vi "WaterVapourSaturationPressure.vi"(1 "Temperature (K)":dbl) -> (0 "Water Vapour Saturation Pressure (Pa)":dbl)   [LabVIEW 2014]
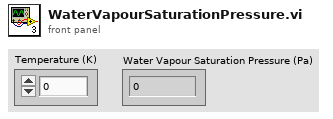
[diagram p1: front panel]
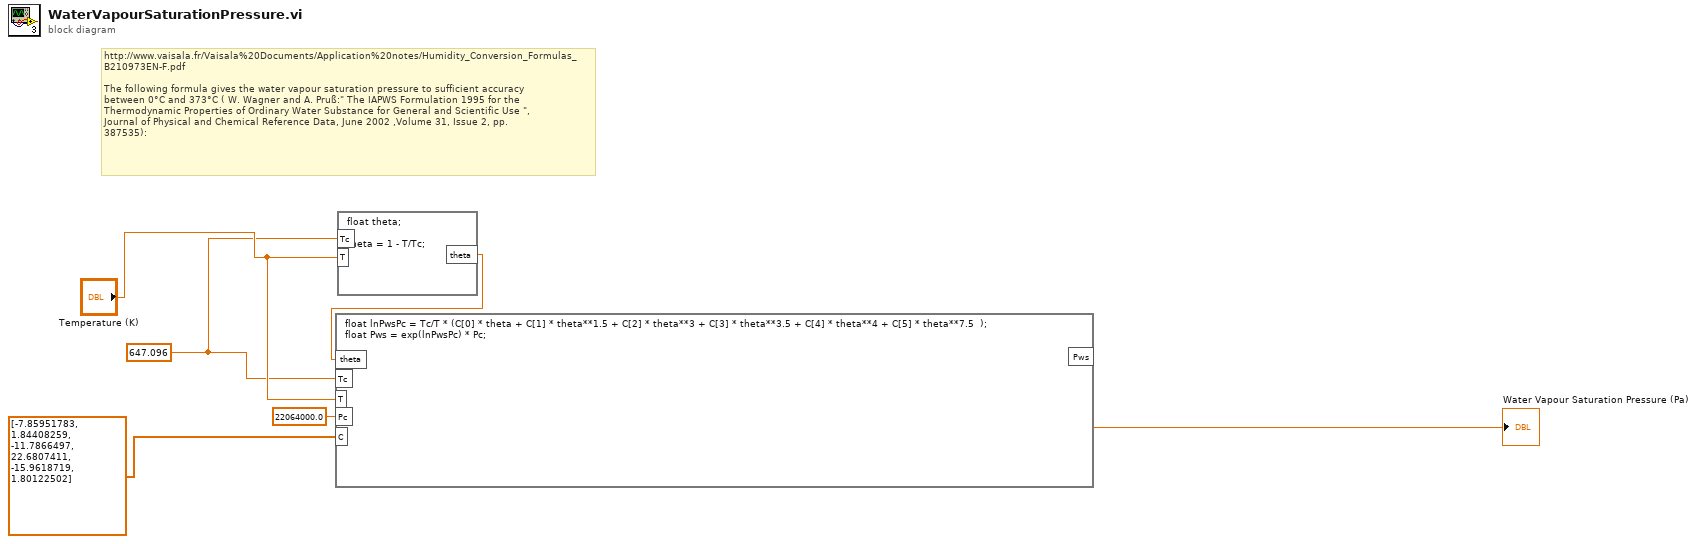
[diagram p0: block diagram]
diagram:
  w1 = 647.096 ("input variable")
  # "http://www.vaisala.fr/Vaisala%20Documents/Application%20notes/Humidity_Conversion_Formulas_B210973EN-F.pdf\n\nThe following formula gives the water vapour saturation pressure to sufficient accuracy\nbetween 0°C and 373°C ( W. Wagner and A. Pruß:\" The IAPWS Formulation 1995 for the\nThermodynamic Properties of Ordinary Water Substance for General and Scientific Use \",\nJournal of Physical and Chemical Reference Data, June 2002 ,Volume 31, Issue 2, pp.\n387535):"
  n1 = formula code="float theta;\n\ntheta = 1 - T/Tc;"("T"="Temperature (K)", "Tc"=w1) -> ("theta"=w4:dbl)
  n2 = formula code="float lnPwsPc = Tc/T * (C[0] * theta + C[1] * theta**1.5 + C[2] * theta**3 + C[3] * theta**3.5 + C[4] * theta**4 + C[5] * theta**7.5  );\nfloat Pws = exp(lnPwsPc) * Pc;"("theta"=w4, "Tc"=w1, "T"="Temperature (K)", "Pc"=22064000.0 ("input variable"), "C"=dbl[] [-7.85951783, 1.84408259, -11.7866497, 22.6807411, -15.9618719, 1.80122502]) -> ("Pws"=→"Water Vapour Saturation Pressure (Pa)":dbl)
